vi "VCS Close All Devices.vi"(8 "error in (no error)":errorcluster) -> (0 "error out":errorcluster)   [LabVIEW 2018]
doc: "<B>VCS Close All Devices</B> closes all opened ports and releases it for other applications."
uses:
  Resources/EposCmd.dll
  Resources/EposCmd64.dll
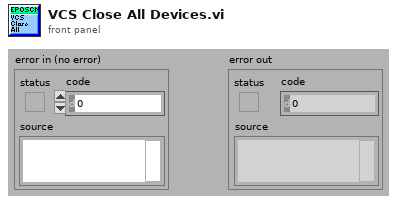
[diagram p1: front panel]
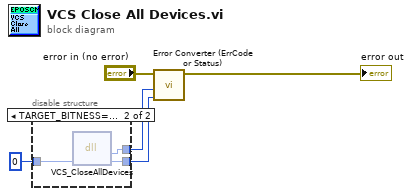
[diagram p0: block diagram]
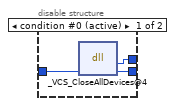
[diagram p2: hidden frame]
diagram:
  n1 = disable-structure shown="TARGET_BITNESS==64" {
    disable-tunnel: u32 0 ("pErrorCode") -> [w8 w11]
    disable-tunnel: [w7 w10] -> w4
    disable-tunnel: [w6 w9] -> w3
    frame condition #0 (active) {
      n2 = dll-call lib="C:/Projeto em LabVIEW/EPOS-LabVIEW-Instrument-Driver-En/LabVIEW/maxon EPOS/Resources/EposCmd.*" fn="_VCS_CloseAllDevices@4"("pErrorCode"=w8) -> (w6:i32, "pErrorCode"=w7:u32)  [unwired: 3 in, 2 out]
    }
    frame condition #1 {
      n3 = dll-call lib="C:/setup/Resources/EposCmd64.dll" fn="VCS_CloseAllDevices" ("EposCmd.dll:_VCS_CloseAllDevices@4")("pErrorCode"=w11) -> ("return type"=w9:i32, "pErrorCode"=w10:u32)  [unwired: 3 in, 2 out]
    }
  }
  n4 = call "Error Converter (ErrCode or Status).vi"("error code"=w4, "return type"=w3, "error in (no error)"="error in (no error)") -> ("error out"=→"error out":errorcluster)  [unwired: 7 in]
